vi "test Secure Client & Server Socket.vi"(8 "error in (no error)":errorcluster, 11 "TestCase in":refnum<class "test Secure Socket.lvclass">) -> (0 "error out":errorcluster, 3 "TestCase out":refnum<class "test Secure Socket.lvclass">)   [LabVIEW 2013, in "test Secure Socket.lvclass"]
uses:
  test Secure Socket.lvclass
  SSL_Lib/SSL-Context/SSL Verify Mode.ctl
  SSL_Lib/SSL-Context/SSL Options.ctl
  SSL_Lib/SSL-Lib/Library Paths.ctl
  SSL Client Context/SSL Client Context.lvclass/SSL Client Context.ctl
  SSL Client Context/SSL Client Context.lvclass
  SSL Client Socket/SSL Client Socket.lvclass
  SSL Server Context/SSL Server Context.lvclass/SSL Server Context.ctl
  SSL Server Context/SSL Server Context.lvclass
  SSL Server Socket/SSL Server Socket.lvclass
  SSL Client Context/Write Verification Options.vi
  SSL Client Context/Write Verification CA Bundle Path.vi
  SSL Client Context/Write SSL Options.vi
  SSL Client Context/Write Cipher List.vi
  SSL Server Context/Write Certificate Chain File.vi
  SSL Server Context/Write Private Key.vi
  <vilib>/addons/_JKI Toolkits/VI Tester/TestCase.llb/TestCase.lvclass
  SSL_Lib/SSL-Context/SSL-Context.lvclass
  SSL_Lib/SSL-Lib/SSL-Lib.lvclass
panel:
  out "Client RX":string
  out "Server RX":string
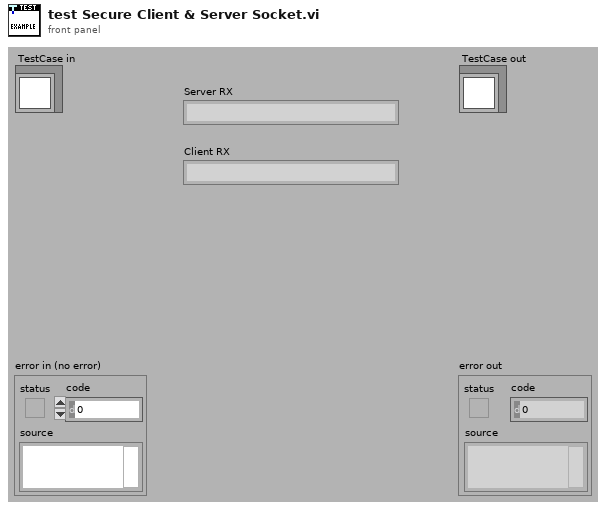
[diagram p1: front panel]
types:
  T1 = typedef "SSL_Lib.lvlib/SSL-Lib.lvclass/Library Paths.ctl" = cluster{"SSL Library Path":path, "Crypto Library Path":path}
  T2 = typedef "SSL_Lib.lvlib/SSL-Context.lvclass/SSL Options.ctl" = i32
  T3 = typedef "SSL_Lib.lvlib/SSL-Context.lvclass/SSL Verify Mode.ctl" = i32
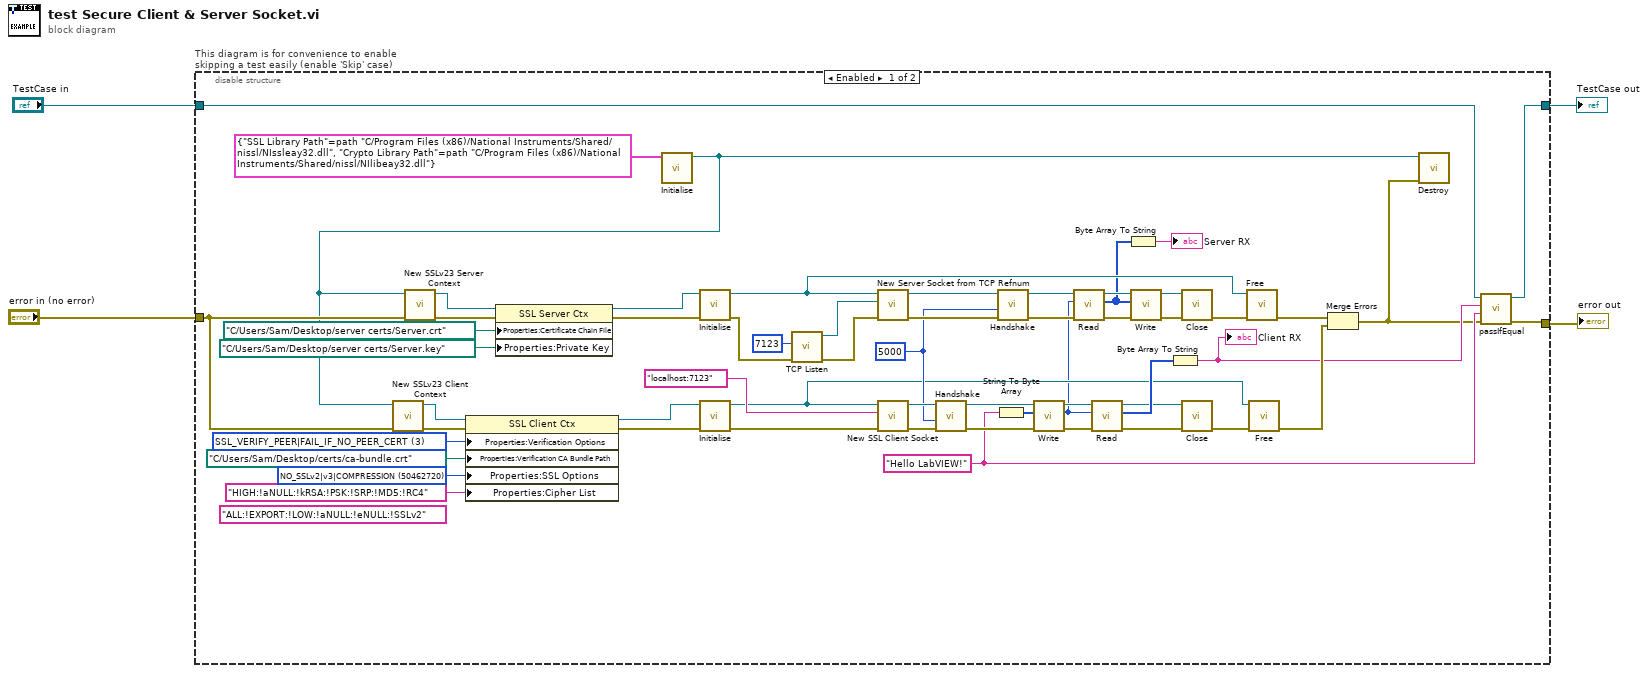
[diagram p0: block diagram]
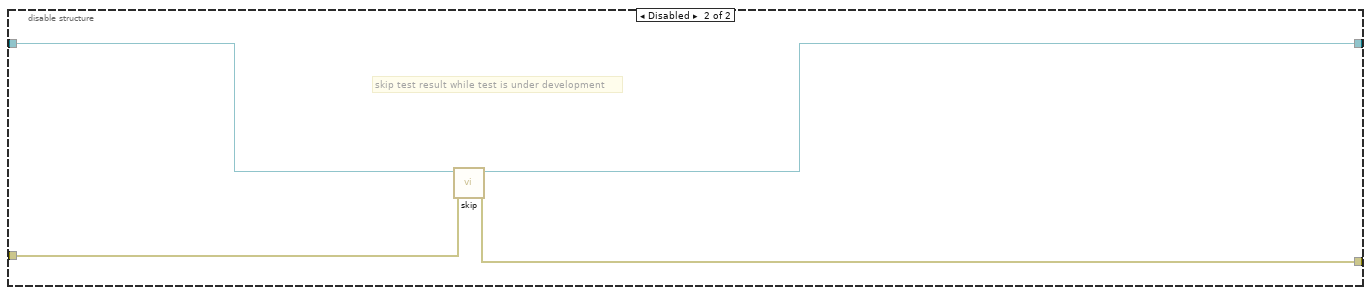
[diagram p2: hidden frame]
diagram:
  n1 = disable-structure "This diagram is for convenience to enable skipping a test easily (enable 'Skip' case)" shown="Enabled" {
    disable-tunnel: "TestCase in" -> [w53 w65]
    disable-tunnel: [w61 w63] -> w1
    disable-tunnel: [w60 w64] -> w3
    disable-tunnel: "error in (no error)" -> [w45 w62]
    frame Enabled {
      w13 = "Hello LabVIEW!"
      w37 = u32 5000 ("Timeout (5000ms)")
      (unwired) "ALL:!EXPORT:!LOW:!aNULL:!eNULL:!SSLv2" ("Cipher List")
      w46 = T2 50462720 items=["None"=0, "NO_SSLv2|v3|COMPRESSION"=50462720, "SSL_OP_NO_COMPRESSION"=131072, "SSL_OP_NO_SSLv2"=16777216, "SSL_OP_NO_SSLv3"=33554432, "SSL_OP_NO_TLSv1"=67108864, "SSL_OP_NO_TLSv1_2"=134217728, "SSL_OP_NO_TLSv1_1"=268435456] ("SSL Options")
      w48 = T3 3 items=["SSL_VERIFY_PEER|FAIL_IF_NO_PEER_CERT"=3, "SSL_VERIFY_NONE"=0, "SSL_VERIFY_PEER"=1, "SSL_VERIFY_FAIL_IF_NO_PEER_CERT"=2, "SSL_VERIFY_CLIENT_ONCE"=4] ("Verification Options")
      n2 = call "Initialise.vi"("Library Paths"=T1 {"SSL Library Path"=path "C:/Program Files (x86)/National Instruments/Shared/nissl/NIssleay32.dll", "Crypto Library Path"=path "C:/Program Files (x86)/National Instruments/Shared/nissl/NIlibeay32.dll"}) -> ("SSL-Lib out"=w6:refnum<class "SSL-Lib.lvclass">)  [unwired: 9 in, 1 out]
      n3 = call "New SSLv23 Client Context.vi"("error in (no error)"=w45, "SSL-Lib"=w6) -> ("error out"=w52:errorcluster, "SSL Client Context out"=w50:refnum<class "SSL Client Context.lvclass">)  [unwired: 8 in]
      n4 = call "New SSLv23 Server Context.vi"("error in (no error)"=w45, "SSL-Lib"=w6) -> ("error out"=w59:errorcluster, "SSL Client Context out"=w57:refnum<class "SSL Server Context.lvclass">)  [unwired: 8 in]
      n5 = property class="SSL Client Ctx"(reference=w50, error in=w52, "Properties:Verification Options"=w48, "Properties:Verification CA Bundle Path"=path "C:/Users/Sam/Desktop/certs/ca-bundle.crt" ("Path to CA bundle"), "Properties:SSL Options"=w46, "Properties:Cipher List"="HIGH:!aNULL:!kRSA:!PSK:!SRP:!MD5:!RC4" ("Cipher List")) -> (reference out=w49:refnum<class "SSL Client Context.lvclass">, error out=w51:errorcluster)
      n6 = property class="SSL Server Ctx"(reference=w57, error in=w59, "Properties:Certificate Chain File"=path "C:/Users/Sam/Desktop/server certs/Server.crt", "Properties:Private Key"=path "C:/Users/Sam/Desktop/server certs/Server.key") -> (reference out=w56:refnum<class "SSL Server Context.lvclass">, error out=w58:errorcluster)
      n7 = call-dynamic "Initialise.vi"("error in (no error)"=w58, "OpenSSL Server Context in"=w56) -> ("error out"=w35:errorcluster, "OpenSSL Server Context out"=w41:refnum<class "SSL Server Context.lvclass">)  [unwired: 8 in]
      n8 = call-dynamic "Initialise.vi"("error in (no error)"=w51, "OpenSSL Client Context in"=w49) -> ("error out"=w38:errorcluster, "OpenSSL Client Context out"=w12:refnum<class "SSL Client Context.lvclass">)  [unwired: 8 in]
      n9 = call <vilib>:"TCP Listen.vi"("error in (no error)"=w35, "port"=u16 7123) -> ("error out"=w34:errorcluster, "connection ID"=w33:refnum<k5>)  [unwired: 5 in, 3 out]
      n10 = call "New Server Socket from TCP Refnum.vi"("error in (no error)"=w34, "TCP Refnum"=w33, "SSL Server Ctx"=w41) -> ("error out"=w42:errorcluster, "SSL Server Skt out"=w43:refnum<class "SSL Server Socket.lvclass">)  [unwired: 7 in]
      n11 = call "New SSL Client Socket.vi"("error in (no error)"=w38, "Hostname / URL"="localhost:7123", "SSL Client Ctx"=w12) -> ("error out"=w39:errorcluster, "SSL Client Skt out"=w40:refnum<class "SSL Client Socket.lvclass">)  [unwired: 7 in]
      n12 = call-dynamic "Handshake.vi"("error in (no error)"=w39, "Timeout (5000ms)"=w37, "OpenSSL in"=w40) -> ("error out"=w31:errorcluster, "OpenSSL out"=w30:refnum<class "SSL Client Socket.lvclass">)  [unwired: 7 in]
      n13 = String To Byte Array(string=w13) -> (unsigned byte array=w24:u8[])
      n14 = call-dynamic "Handshake.vi"("error in (no error)"=w42, "Timeout (5000ms)"=w37, "OpenSSL in"=w43) -> ("error out"=w28:errorcluster, "OpenSSL out"=w29:refnum<class "SSL Server Socket.lvclass">)  [unwired: 7 in]
      n15 = call-dynamic "Write.vi"("error in (no error)"=w31, "Bytes to write"=w24, "OpenSSL Socket in"=w30) -> ("error out"=w23:errorcluster, "bytes written"=w11:i32, "OpenSSL Socket out"=w27:refnum<class "SSL Client Socket.lvclass">)  [unwired: 6 in]
      n16 = call-dynamic "Read.vi"("error in (no error)"=w28, "# bytes to read"=w11, "OpenSSL Socket in"=w29) -> ("error out"=w26:errorcluster, "Read Bytes"=w10:u8[], "OpenSSL Socket out"=w25:refnum<class "SSL Server Socket.lvclass">)  [unwired: 6 in]
      n17 = call-dynamic "Read.vi"("error in (no error)"=w23, "# bytes to read"=w11, "OpenSSL Socket in"=w27) -> ("error out"=w8:errorcluster, "Read Bytes"=w22:u8[], "OpenSSL Socket out"=w20:refnum<class "SSL Client Socket.lvclass">)  [unwired: 6 in]
      n18 = Byte Array To String(unsigned byte array=w10) -> (string=→"Server RX":string)
      n19 = call-dynamic "Write.vi"("error in (no error)"=w26, "Bytes to write"=w10, "OpenSSL Socket in"=w25) -> ("error out"=w19:errorcluster, "OpenSSL Socket out"=w18:refnum<class "SSL Server Socket.lvclass">)  [unwired: 6 in, 1 out]
      n20 = Byte Array To String(unsigned byte array=w22) -> (string=w14:string)
      "Client RX" <- w14
      n21 = call-dynamic "Close.vi"("error in (no error)"=w19, "OpenSSL Socket in"=w18) -> ("error out"=w17:errorcluster)  [unwired: 9 in]
      n22 = call-dynamic "Close.vi"("error in (no error)"=w8, "OpenSSL Socket in"=w20) -> ("error out"=w21:errorcluster)  [unwired: 9 in]
      n23 = call-dynamic "Free.vi"("error in (no error)"=w17, "OpenSSL Context in"=w41) -> ("error out"=w16:errorcluster)  [unwired: 9 in]
      n24 = call-dynamic "Free.vi"("error in (no error)"=w21, "OpenSSL Context in"=w12) -> ("error out"=w15:errorcluster)  [unwired: 9 in]
      n25 = Merge Errors(w16, w15) -> (w5:errorcluster)
      n26 = call "Destroy.vi"("error in (no error)"=w5, "SSL-Lib in"=w6) -> ()  [unwired: 9 in, 1 out]
      n27 = call-dynamic "passIfEqual.vi"("error in (no error)"=w5, "y"=w13, "x"=w14, "TestCase in"=w53) -> ("error out"=w60:errorcluster, "TestCase out"=w61:refnum<class "test Secure Socket.lvclass">)  [unwired: 6 in]
    }
    frame Disabled {
      # "skip test result while test is under development"
      n28 = call <vilib>:"skip.vi"("error in (no error)"=w62, "TestCase in"=w65) -> ("error out"=w64:errorcluster, "TestCase out"=w63:refnum<class "test Secure Socket.lvclass">)  [unwired: 8 in]
    }
  }
  "error out" <- w3
  "TestCase out" <- w1
